vi "Shutdown.vi"(8 "error in (no error)":errorcluster, 11 "DemoCamera in":refnum<class "DemoCamera.lvclass">) -> (0 "error out":errorcluster, 3 "DemoCamera out":refnum<class "DemoCamera.lvclass">)   [LabVIEW 2020, in "DemoCamera.lvlib" / "DemoCamera.lvclass"]
uses:
  DemoCamera.lvclass
  Hardware Abstraction Layer/Component/Camera/Camera/Camera.lvclass
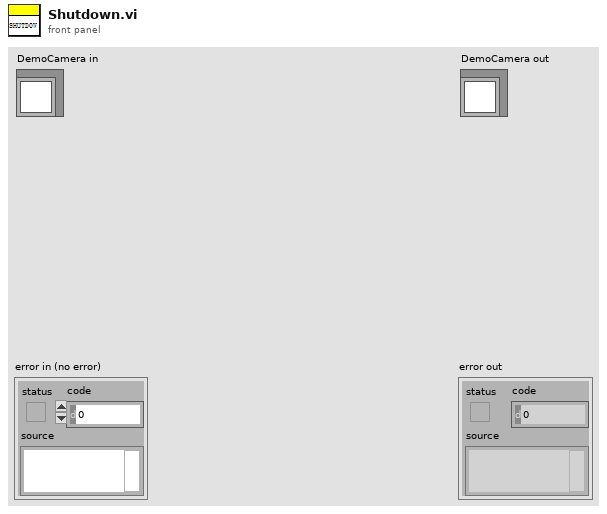
[diagram p1: front panel]
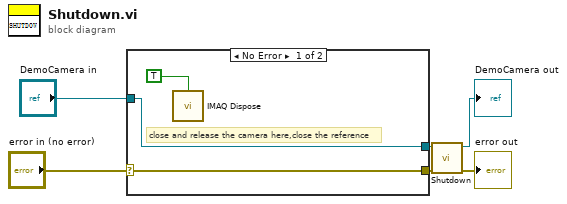
[diagram p0: block diagram]
diagram:
  n1 = case shown="No Error" "error in (no error)" {
    selector: "error in (no error)" -> [w9 w10]
    tunnel: [w9 w10] -> w4
    tunnel: "DemoCamera in" -> [w8 w11]
    tunnel: [w8 w11] -> w1
    frame No Error {
      # "close and release the camera here,close the reference"
      n2 = call "IMAQ Dispose"("All Images? (No)"=TRUE) -> ()  [unwired: 5 in, 1 out]
    }
    frame Error {
    }
  }
  n3 = call-parent "Shutdown.vi"("error in (no error)"=w4, "Device in"=w1) -> ("error out"=→"error out":errorcluster, "Device out"=→"DemoCamera out":refnum<class "DemoCamera.lvclass">)  [unwired: 8 in]
